vi "dosimat876_volume_query.vi"(0 "error in":errorcluster, 1 "Dosimat Port In":refnum<visa-resource-name>="COM1") -> (2 "error out":errorcluster, 3 "Volume":dbl, 4 "Dosimat Port Out":refnum<visa-resource-name>="COM1")   [LabVIEW 2010]
panel:
  out "first string return":string
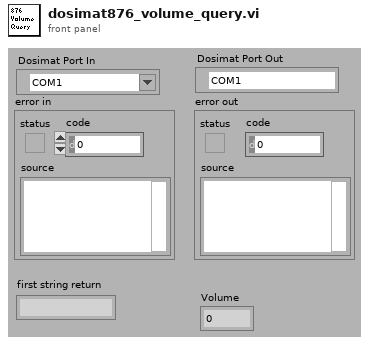
[diagram p1: front panel]
types:
  T1 = cluster{"Dosimat Port out":refnum<visa-resource-name>, "Error out":errorcluster}
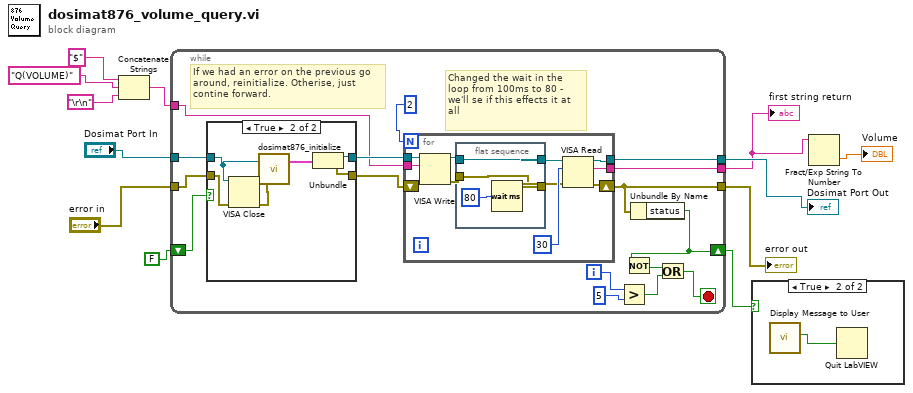
[diagram p0: block diagram]
diagram:
  n1 = Concatenate Strings("$" ("string"), "Q(VOLUME)" ("Method"), "\r\n") -> (w6:string)
  n2 = while {
    tunnel: "Dosimat Port In" -> [w17]
    tunnel: "error in" -> [w14]
    tunnel: w6 -> [w16]
    tunnel: [w28] -> w5
    tunnel: [w25] -> w4
    tunnel: [w27] -> w3
    shift-right: [w19] -> w2
    shift-left: FALSE -> [w13]
    i -> [w22]
    stop <- w20 stop-if-true
    # "If we had an error on the previous go around, reinitialize. Otherise, just contine forward."
    # "Changed the wait in the loop from 100ms to 80 - we'll se if this effects it at all"
    n3 = case shown="True" w13 {
      tunnel: [w30 w35] -> w18
      tunnel: w17 -> [w30 w33]
      tunnel: [w29 w34] -> w15
      tunnel: w14 -> [w29 w32]
      frame False {
      }
      frame True {
        n4 = VISA Close(VISA resource name=w33, error in (no error)=w32) -> (error out=w31:errorcluster)
        n5 = call "dosimat876_initialize.vi"("error in"=w31, "Dosimat Port In"=w33) -> ("Dosimat Out"=w36:T1)  [unwired: 1 in]
        n6 = Unbundle(w36) -> ("Dosimat Port out"=w35:refnum<visa-resource-name>, "Error out"=w34:errorcluster)
      }
    }
    n7 = for {
      N: 2 -> [_]
      tunnel: w18 -> [w46]
      tunnel: w16 -> [w44]
      tunnel: [w43] -> w28
      tunnel: [w41] -> w27
      shift-right: [w42] -> w25
      shift-left: w15 -> [w45]
      n8 = VISA Write(VISA resource name=w46, write buffer=w44, error in (no error)=w45) -> (VISA resource name out=w37:refnum<visa-resource-name>, error out=w39:errorcluster)  [unwired: 1 out]
      n9 = flat-sequence {
        tunnel: [w50] -> w40
        tunnel: w39 -> [w50]
        tunnel: [w49] -> w38
        tunnel: w37 -> [w49]
        frame #0 {
          n10 = Wait (ms)(milliseconds to wait=80) -> ()  [unwired: 1 out]
        }
      }
      n11 = VISA Read(VISA resource name=w38, byte count=u32 30, error in (no error)=w40) -> (VISA resource name out=w43:refnum<visa-resource-name>, read buffer=w41:string, error out=w42:errorcluster)  [unwired: 1 out]
    }
    n12 = Greater?(x=w22, y=5) -> (0:w21:bool)
    n13 = Unbundle By Name(w25) -> ("status"=w19:bool)
    n14 = Not(x=w19) -> (.not. x?=w24:bool)
    n15 = Or(x=w24, y=w21) -> (x .or. y?=w20:bool)
  }
  "Dosimat Port Out" <- w5
  "error out" <- w4
  "first string return" <- w3
  n16 = case shown="True" w2 {
    frame False {
    }
    frame True {
      n17 = call "Display Message to User"() -> ("OK"=w51:bool)  [unwired: 10 in, 1 out]
      n18 = Quit LabVIEW(quit? (T)=w51) -> ()
    }
  }
  n19 = Fract/Exp String To Number(string=w3) -> (number=→"Volume":dbl)  [unwired: 3 in, 1 out]
